vi "BS set the camera.vi"(2 "error in":errorcluster, 3 "IMAQdx Session input":T1) -> (0 "error out":errorcluster, 1 "IMAQdx Session output":T1)   [LabVIEW 2012]
doc: "This VI sets the camera values for the Point Grey Grasshopper camera above the pool for the final Robotics I Final Project."
uses:
  <vilib>/userdefined/High Color/IMAQdx.ctl
  <resource>/objmgr/imaqdx.rc
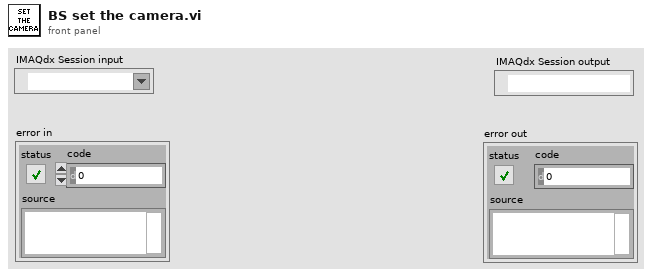
[diagram p1: front panel]
types:
  T1 = typedef "IMAQdx.ctl" = refnum<k21>
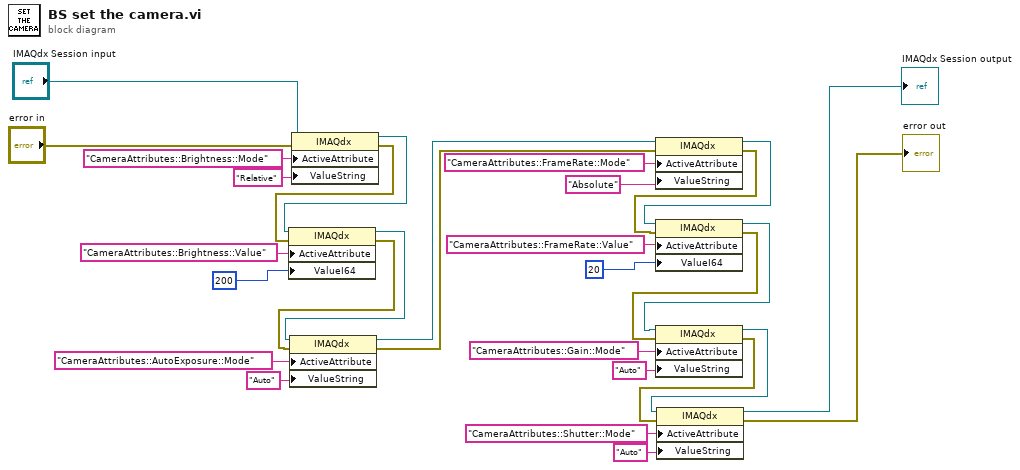
[diagram p0: block diagram]
diagram:
  n1 = property class="IMAQdx"(reference="IMAQdx Session input", error in="error in", "ActiveAttribute"="CameraAttributes::Brightness::Mode", "ValueString"="Relative") -> (reference out=w29:T1, error out=w7:errorcluster)
  n2 = property class="IMAQdx"(reference=w29, error in=w7, "ActiveAttribute"="CameraAttributes::Brightness::Value", "ValueI64"=i64 200 ("Brightness")) -> (reference out=w21:T1, error out=w6:errorcluster)
  n3 = property class="IMAQdx"(reference=w21, error in=w6, "ActiveAttribute"="CameraAttributes::AutoExposure::Mode", "ValueString"="Auto") -> (reference out=w20:T1, error out=w5:errorcluster)
  n4 = property class="IMAQdx"(reference=w20, error in=w5, "ActiveAttribute"="CameraAttributes::FrameRate::Mode", "ValueString"="Absolute") -> (reference out=w16:T1, error out=w4:errorcluster)
  n5 = property class="IMAQdx"(reference=w16, error in=w4, "ActiveAttribute"="CameraAttributes::FrameRate::Value", "ValueI64"=i64 20 ("Frame Rate")) -> (reference out=w13:T1, error out=w3:errorcluster)
  n6 = property class="IMAQdx"(reference=w13, error in=w3, "ActiveAttribute"="CameraAttributes::Gain::Mode", "ValueString"="Auto") -> (reference out=w11:T1, error out=w2:errorcluster)
  n7 = property class="IMAQdx"(reference=w11, error in=w2, "ActiveAttribute"="CameraAttributes::Shutter::Mode", "ValueString"="Auto") -> (reference out=→"IMAQdx Session output":T1, error out=→"error out":errorcluster)
